vi "Progress Popup Example.vi"   [LabVIEW 2020]
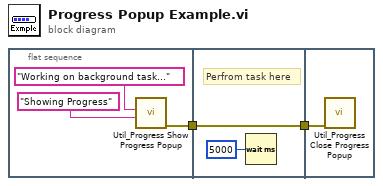
[diagram p0: block diagram]
diagram:
  n1 = flat-sequence {
    tunnel: [w3] -> w1
    tunnel: [w6] -> w2
    tunnel: w1 -> [w6]
    tunnel: w2 -> [w8]
    frame #0 {
      n2 = call "Util_Progress Show Progress Popup.vi"("Title"="Showing Progress" ("Process Progress"), "Message"="Working on background task...") -> ("error out"=w3:errorcluster)  [unwired: 9 in]
    }
    frame #1 {
      # "Perfrom task here"
      n3 = Wait (ms)(milliseconds to wait=u32 5000 ("millisecond multiple")) -> ()  [unwired: 1 out]
    }
    frame #2 {
      n4 = call "Util_Progress Close Progress Popup.vi"("error in (no error)"=w8) -> ()  [unwired: 10 in, 1 out]
    }
  }
